vi "F1.vi"(8 "s":dbl, 9 "d":dbl, 10 "w":dbl, 11 "a":dbl) -> (2 "F1":dbl format="%#_13g")   [LabVIEW 2021]
panel:
  out "Array":dbl[](array[numeric])
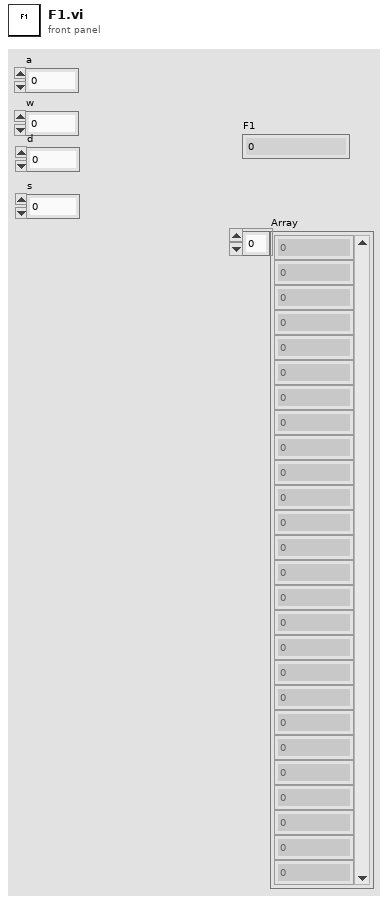
[diagram p1: front panel]
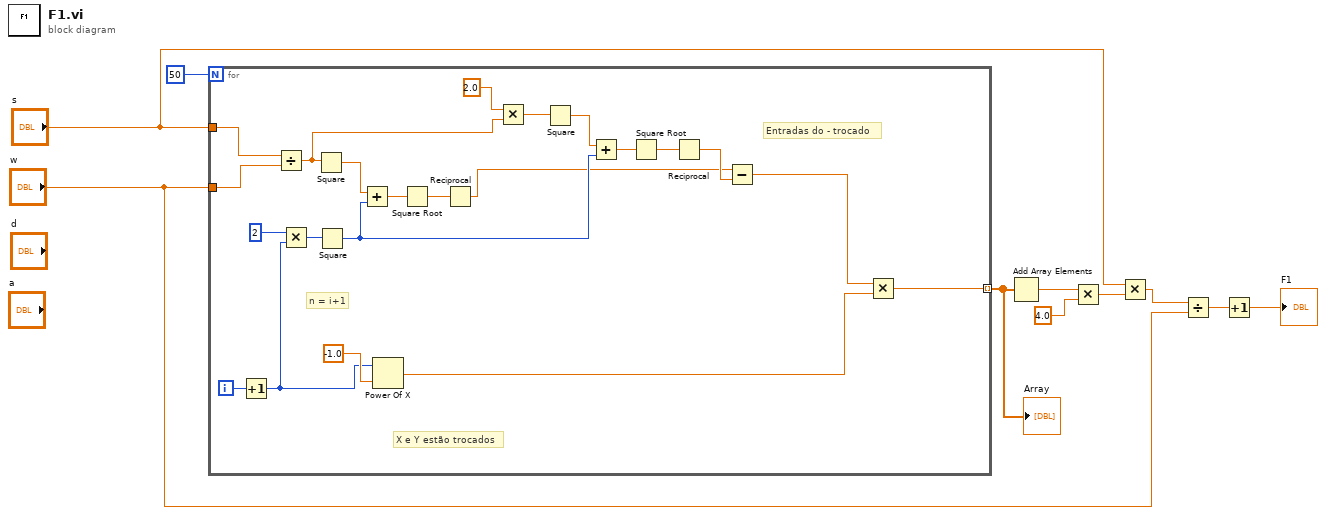
[diagram p0: block diagram]
diagram:
  n1 = for {
    N: 50 -> [_]
    tunnel: "s" -> [w31]
    tunnel: "w" -> [w30]
    tunnel: [w17] -> w10 mode=indexing
    i -> [w15]
    # "n = i+1"
    # "Entradas do - trocado"
    # "X e Y estão trocados"
    n2 = Increment(x=w15) -> (x+1=w13:i32)
    n3 = Divide(x=w31, y=w30) -> (x/y=w19:dbl)
    n4 = Multiply(x=2, y=w13) -> (x*y=w28:i32)
    n5 = Square(x=w19) -> (x^2=w27:dbl)
    n6 = Square(x=w28) -> (x^2=w22:i32)
    n7 = Add(x=w27, y=w22) -> (x+y=w26:dbl)
    n8 = Power Of X(1:-1.0 ("y"), 2:w13) -> (0:w16:dbl)
    n9 = Square Root(x=w26) -> (sqrt(x)=w32:dbl)
    n10 = Reciprocal(x=w32) -> (1/x=w11:dbl)
    n11 = Multiply(x=2.0, y=w19) -> (x*y=w21:dbl)
    n12 = Square(x=w21) -> (x^2=w24:dbl)
    n13 = Add(x=w24, y=w22) -> (x+y=w23:dbl)
    n14 = Square Root(x=w23) -> (sqrt(x)=w25:dbl)
    n15 = Reciprocal(x=w25) -> (1/x=w12:dbl)
    n16 = Subtract(x=w11, y=w12) -> (x-y=w18:dbl)
    n17 = Multiply(x=w18, y=w16) -> (x*y=w17:dbl)
  }
  "Array" <- w10
  n18 = Add Array Elements(numeric array=w10) -> (sum=w9:dbl)
  n19 = Multiply(x=w9, y=4.0) -> (x*y=w7:dbl)
  n20 = Multiply(x="s", y=w7) -> (x*y=w5:dbl)
  n21 = Divide(x=w5, y="w") -> (x/y=w3:dbl)
  n22 = Increment(x=w3) -> (x+1=→"F1":dbl)
